vi "poly_detect_boolean_edges_both.vi"(4 "tf input":bool) -> (1 "edge":bool)   [LabVIEW 2015]
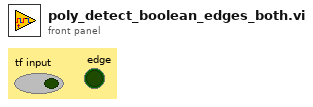
[diagram p1: front panel]
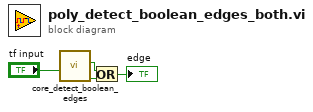
[diagram p0: block diagram]
diagram:
  n1 = call "core_detect_boolean_edges.vi"("tf input"="tf input") -> ("falling edge"=w2:bool, "rising edge"=w3:bool)  [unwired: 9 in]
  n2 = Or(x=w3, y=w2) -> (x .or. y?=→"edge":bool)
